vi "qp_AS evaluate feasibility.vi"(4 "b":dbl[](array[numeric]), 5 "Xmax":dbl[](array[numeric]), 6 "A":dbl[][](array[numeric]), 7 "Xmin":dbl[](array[numeric]), 8 "Imax":dbl[](array[numeric]), 9 "Imin":dbl[](array[numeric]), 10 "D":dbl[][](array[numeric]), 11 "X":dbl[](array[numeric])) -> (3 "feasible?":bool)   [LabVIEW 2018, in "NI_Gmath.lvlib"]
uses:
  NI_Gmath.lvlib
  A x Vector.vi
  <vilib>/Analysis/NI_AALBase.lvlib
panel:
  in  "tolerance":dbl=1e-06
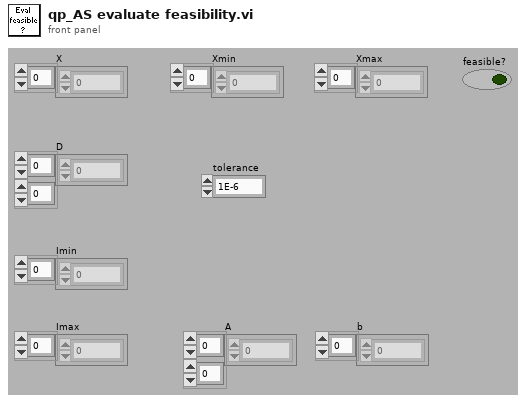
[diagram p1: front panel]
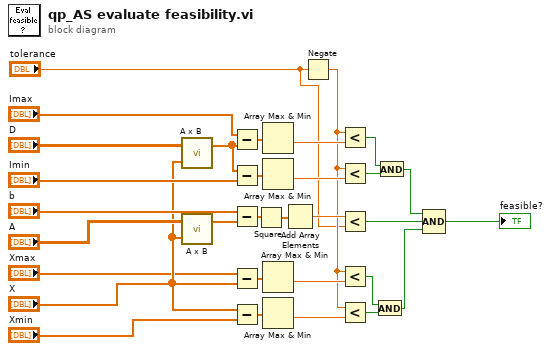
[diagram p0: block diagram]
diagram:
  n1 = call-poly "A x B.vi"("Vector"="X", "A"="D") -> ("A x Vector"=w6:dbl[])  [unwired: 1 out]
  n2 = call-poly "A x B.vi"("Vector"="X", "A"="A") -> ("A x Vector"=w22:dbl[])  [unwired: 1 out]
  n3 = Subtract(x="Imax", y=w6) -> (x-y=w7:dbl[])
  n4 = Subtract(x=w6, y="Imin") -> (x-y=w8:dbl[])
  n5 = Subtract ("Subtract.vi")(x="b", y=w22) -> (x-y=w21:dbl[])
  n6 = Subtract(x="Xmax", y="X") -> (x-y=w18:dbl[])
  n7 = Subtract(x="X", y="Xmin") -> (x-y=w17:dbl[])
  n8 = Square(x=w21) -> (x^2=w20:dbl[])
  n9 = Array Max & Min(array=w7) -> (min value=w9:dbl)  [unwired: 3 out]
  n10 = Array Max & Min(array=w8) -> (min value=w10:dbl)  [unwired: 3 out]
  n11 = Array Max & Min(array=w18) -> (min value=w16:dbl)  [unwired: 3 out]
  n12 = Array Max & Min(array=w17) -> (min value=w15:dbl)  [unwired: 3 out]
  n13 = Add Array Elements(numeric array=w20) -> (sum=w19:dbl)
  n14 = Negate(x="tolerance") -> (-x=w2:dbl)
  n15 = Less?(x=w2, y=w9) -> (x < y?=w11:bool)
  n16 = Less?(x=w2, y=w10) -> (x < y?=w12:bool)
  n17 = Less?(x=w19, y="tolerance") -> (x < y?=w4:bool)
  n18 = Less?(x=w2, y=w16) -> (x < y?=w14:bool)
  n19 = Less?(x=w2, y=w15) -> (x < y?=w13:bool)
  n20 = And(x=w14, y=w13) -> (x .and. y?=w3:bool)
  n21 = And(x=w11, y=w12) -> (x .and. y?=w5:bool)
  n22 = Compound Arithmetic op=AND(w5, w4, w3) -> (→"feasible?":bool)
